vi "Write SwitchACIR Channel.vi"(8 "error in (no error)":errorcluster, 10 "SwitchACIR Channel":T1, 11 "ACIR configuration":refnum<class "SwitchACIR Channel configuration.lvclass">) -> (0 "error out":errorcluster, 3 "ACIR configuration out":refnum<class "SwitchACIR Channel configuration.lvclass">)   [LabVIEW 2025, in "SwitchACIR Channel configuration.lvclass"]
uses:
  SwitchACIR Channel configuration.lvclass
  SwitchACIR Channel Setting.ctl
  SwitchACIR Channel configuration.lvclass/SwitchACIR Channel configuration.ctl
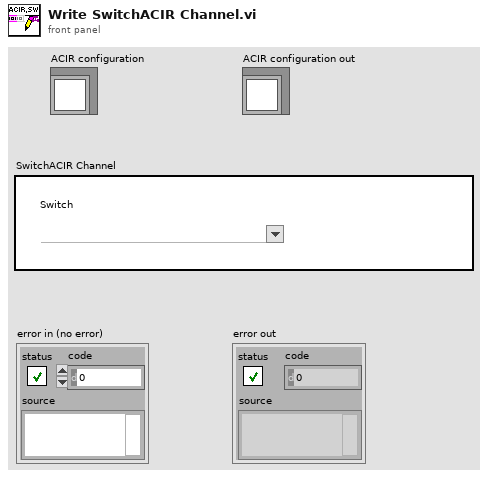
[diagram p1: front panel]
types:
  T1 = typedef "SwitchACIR Channel configuration.lvclass/SwitchACIR Channel Setting.ctl" = cluster{"Switch":string}
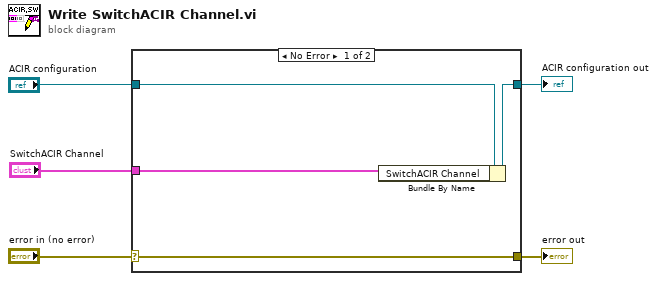
[diagram p0: block diagram]
diagram:
  n1 = case shown="No Error" "error in (no error)" {
    selector: "error in (no error)" -> [w9 w10]
    tunnel: [w9 w10] -> w4
    tunnel: [w7 w11] -> w2
    tunnel: "ACIR configuration" -> [w8 w11]
    tunnel: "SwitchACIR Channel" -> [w6 _]
    frame No Error {
      n2 = Bundle By Name(cluster=w8, "SwitchACIR Channel"=w6) -> (w7:refnum<class "SwitchACIR Channel configuration.lvclass">)
    }
    frame Error {
    }
  }
  "error out" <- w4
  "ACIR configuration out" <- w2
